vi "Hold Position.vi"() -> (2 "Holding Position":dbl)   [LabVIEW 2017]
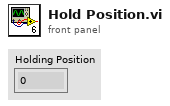
[diagram p1: front panel]
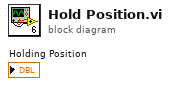
[diagram p0: block diagram]
diagram:
